vi "Set Pixel clock.vi"(11 "Refresh":bool) -> ()   [LabVIEW 2015]
uses:
  <vilib>/rvi/Emulation/niFpgaSctlEmulationGetInTimedLoop.vi
  Globals/Global Variable_Pixel Clock.vi
  <vilib>/rvi/Emulation/niFpgaProcessEmulError.vi
  <vilib>/rvi/eio/common/nirviEmuTemplateMethod_errors.vi
  <vilib>/eio/EIONode/EIONode.xnode
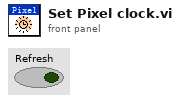
[diagram p1: front panel]
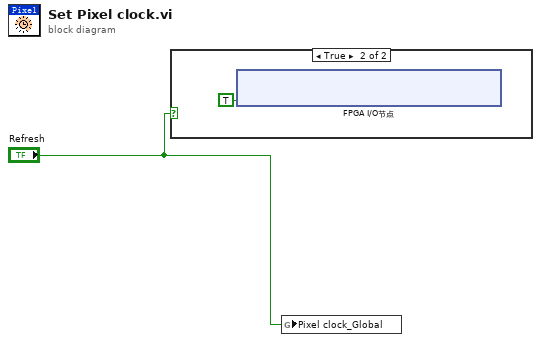
[diagram p0: block diagram]
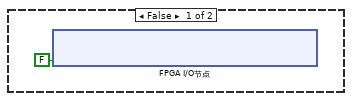
[diagram p2: hidden frame]
diagram:
  n1 = case shown="True" "Refresh" {
    frame False {
      n2 = xnode "FPGA I/O节点"("IO Module\\(Pixel clock)DDCB_PFI3_WRITE"=FALSE ("IO Module\\(Pixel clock)DDCB_PFI3_WRITE")) -> ()  [unwired: 1 in, 1 out]
    }
    frame True {
      n3 = xnode "FPGA I/O节点"("IO Module\\(Pixel clock)DDCB_PFI3_WRITE"=TRUE ("IO Module\\(Pixel clock)DDCB_PFI3_WRITE")) -> ()  [unwired: 1 in, 1 out]
    }
  }
  n4 = global write "Global Variable_Pixel Clock.vi" "Pixel clock_Global"("Refresh") -> ()
